vi "Get Fiducials.vi"(6 "error in":errorcluster, 7 "Image Prefix":string, 8 "Fiducial Type":string, 9 "CameraTool In":refnum<class "CameraTool Class.lvclass">=refnum) -> (0 "error out":errorcluster, 1 "Fiducial Image":T1, 2 "Fiducial Image Positions":refnum<class "Vec3d.lvclass">[](array[class]), 3 "CameraTool Out":refnum<class "CameraTool Class.lvclass">)   [LabVIEW 2017, in "CameraTool Class.lvclass"]
doc: "This VI looks for fiducials in input images. It returns the number of fiducials found in the input image and a list of up to 10 x,y pairs of fiducial locations in the image.\n\nImage Name can be given if multiple images are wanted to be collected. Otherwise, the image must be disposed of before calling again."
uses:
  CameraTool Class.lvclass
  Vec3d Class/Vec3d.lvclass
  <vilib>/vision/Image Controls.llb/IMAQ Image.ctl
  Utils/Type Definitions/Physical Image.ctl
  FlexWorktable/FlexWorktable.lvclass
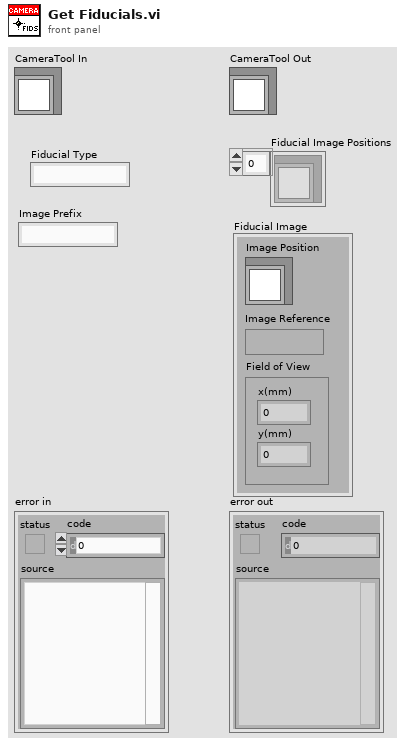
[diagram p1: front panel]
types:
  T1 = typedef "Physical Image.ctl" = cluster{"Image Position":refnum<class "Vec3d.lvclass">, "Image Reference":T2, "Field of View":cluster{"x(mm)":dbl, "y(mm)":dbl}}
  T2 = typedef "IMAQ Image.ctl" = refnum<image>
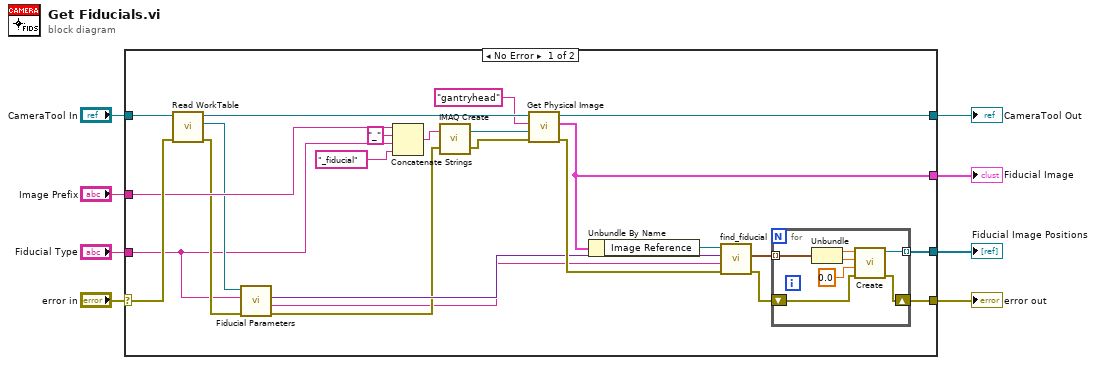
[diagram p0: block diagram]
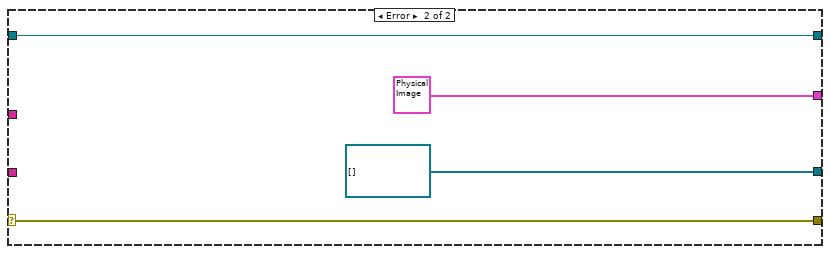
[diagram p2: hidden frame]
diagram:
  n1 = case shown="No Error" "error in" {
    selector: "error in" -> [w32 w43]
    tunnel: [w29 w43] -> w7
    tunnel: "CameraTool In" -> [w26 w42]
    tunnel: [w31 w42] -> w5
    tunnel: [w30 refnum<class "Vec3d.lvclass">[] []] -> w4
    tunnel: [w28 T1 {"Image Position"=refnum, "Image Reference"=refnum, "Field of View"={"x(mm)"=0.0, "y(mm)"=0.0}} ("Physical Image")] -> w3
    tunnel: "Image Prefix" -> [w27 _]
    tunnel: "Fiducial Type" -> [w9 _]
    frame No Error {
      n2 = call-dynamic "Read WorkTable.vi"("error in"=w32, "Gantry Class in"=w26) -> ("error out"=w12:errorcluster, "Worktable"=w13:refnum<class "FlexWorktable.lvclass">, "Gantry Class out"=w25:refnum<class "CameraTool Class.lvclass">)  [unwired: 7 in]
      n3 = call-dynamic "Fiducial Parameters.vi"("error in (no error)"=w12, "Fiducial Type"=w9, "FlexWorktable in"=w13) -> ("error out"=w11:errorcluster, "Fiducial Method"=w10:string, "Fiducial Parameters"=w14:variant)  [unwired: 4 in, 2 out]
      n4 = Concatenate Strings(w27, "_" ("string"), w9, "_fiducial" ("string")) -> (w19:string)
      n5 = call "IMAQ Create"("Image Name"=w19, "error in (no error)"=w11) -> ("New Image"=w21:T2, "error out"=w16:errorcluster)  [unwired: 3 in]
      n6 = call-dynamic "Get Physical Image.vi"("error in"=w16, "Image In"=w21, "Camera Name"="gantryhead", "Gantry in"=w25) -> ("error out"=w23:errorcluster, "Physical Image"=w28:T1, "Gantry out"=w31:refnum<class "CameraTool Class.lvclass">)  [unwired: 5 in]
      n7 = Unbundle By Name(w28) -> ("Image Reference"=w20:T2)
      n8 = call "find_fiducial.vi"("error in"=w23, "interactive"=w10, "Fiducial Parameters"=w14, "Image"=w20) -> ("error out"=w24:errorcluster, "coords"=w22:cluster{"x":dbl, "y":dbl}[])  [unwired: 6 in]
      n9 = for {
        tunnel: [w39] -> w30 mode=indexing
        shift-right: [w37] -> w29
        shift-left: w24 -> [w38]
        tunnel: w22 -> [w35] mode=indexing
        n10 = Unbundle(w35) -> ("x"=w34:dbl, "y"=w33:dbl)
        n11 = call "Create.vi"("error in"=w38, "Z"=0.0, "Y"=w33, "X"=w34) -> ("error out"=w37:errorcluster, "Vec3d Class out"=w39:refnum<class "Vec3d.lvclass">)  [unwired: 6 in]
      }
    }
    frame Error {
    }
  }
  "error out" <- w7
  "CameraTool Out" <- w5
  "Fiducial Image Positions" <- w4
  "Fiducial Image" <- w3
